vi "GenerateDigital.vi"   [LabVIEW 2013]
uses:
  C:/Program Files (x86)/LabNation/SmartScope/DeviceInterface.dll
  Program Files (x86)/LabNation/SmartScope/DeviceInterface.dll
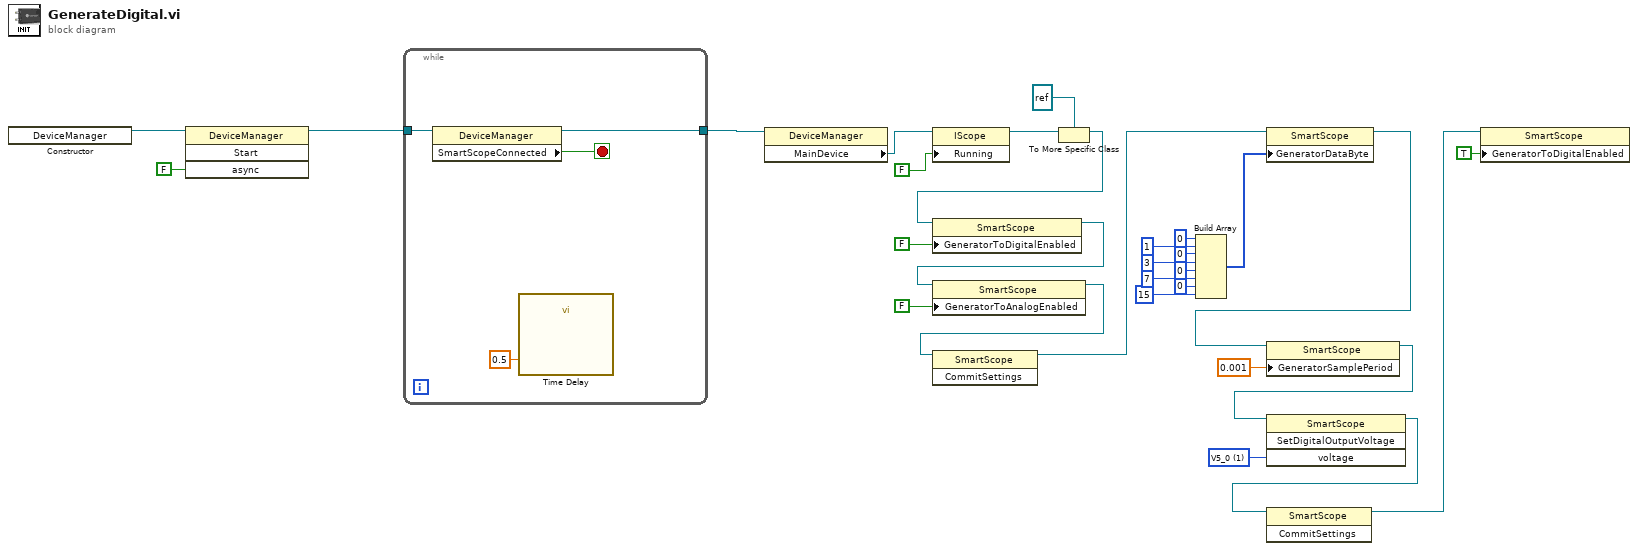
[diagram p0: block diagram]
diagram:
  w7 = 1 items=["V3_0", "V5_0"] ("voltage")
  n1 = constructor class="DeviceManager"() -> (reference out=w26:refnum<k24>)  [unwired: 3 in, 2 out]
  n2 = invoke class="DeviceManager" method="Start"(reference=w26, "async"=FALSE) -> (reference out=w27:refnum<k24>)  [unwired: 2 in, 3 out]
  n3 = while {
    tunnel: w27 -> [w33]
    tunnel: [w32] -> w29
    stop <- w31 stop-if-true
    n4 = property class="DeviceManager"(reference=w33) -> (reference out=w32:refnum<k24>, "SmartScopeConnected"=w31:bool)  [unwired: 1 in, 1 out]
    n5 = call "Time Delay"("Delay Time (s)"=0.5) -> ()  [unwired: 10 in, 1 out]
  }
  n6 = property class="DeviceManager"(reference=w29) -> ("MainDevice"=w2:refnum<k24>)  [unwired: 1 in, 2 out]
  n7 = property class="IScope"(reference=w2, "Running"=FALSE) -> (reference out=w23:refnum<k24>)  [unwired: 1 in, 1 out]
  n8 = To More Specific Class(target class=refnum<k24> refnum, reference=w23) -> (specific class reference=w21:refnum<k24>)  [unwired: 1 in, 1 out]
  n9 = property class="SmartScope"(reference=w21, "GeneratorToDigitalEnabled"=FALSE) -> (reference out=w20:refnum<k24>)  [unwired: 1 in, 1 out]
  n10 = property class="SmartScope"(reference=w20, "GeneratorToAnalogEnabled"=FALSE ("GeneratorToDigitalEnabled")) -> (reference out=w1:refnum<k24>)  [unwired: 1 in, 1 out]
  n11 = invoke class="SmartScope" method="CommitSettings"(reference=w1) -> (reference out=w9:refnum<k24>)  [unwired: 2 in, 2 out]
  n12 = Build Array(u8 0 ("element"), u8 1 ("element"), u8 0 ("element"), u8 3 ("element"), u8 0 ("element"), u8 7 ("element"), u8 0 ("element"), u8 15 ("element")) -> (w19:u8[])
  n13 = property class="SmartScope"(reference=w9, "GeneratorDataByte"=w19) -> (reference out=w8:refnum<k24>)  [unwired: 1 in, 1 out]
  n14 = property class="SmartScope"(reference=w8, "GeneratorSamplePeriod"=0.001) -> (reference out=w6:refnum<k24>)  [unwired: 1 in, 1 out]
  n15 = invoke class="SmartScope" method="SetDigitalOutputVoltage"(reference=w6, "voltage"=w7) -> (reference out=w5:refnum<k24>)  [unwired: 2 in, 3 out]
  n16 = invoke class="SmartScope" method="CommitSettings"(reference=w5) -> (reference out=w3:refnum<k24>)  [unwired: 2 in, 2 out]
  n17 = property class="SmartScope"(reference=w3, "GeneratorToDigitalEnabled"=TRUE) -> ()  [unwired: 1 in, 2 out]
